vi "cal_p.vi"() -> ()   [LabVIEW 2013]
panel:
  in  "c":dbl
  in  "b":dbl=1.0
  in  "a":dbl
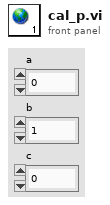
[diagram p1: front panel]
diagram:
